vi "RFSA Configure Trigger.vi"(8 "error in (no error)":errorcluster, 11 "IVI Refnum in":refnum<k15>) -> (0 "error out":errorcluster, 3 "IVI Refnum out":refnum<k15>)   [LabVIEW 2021]
uses:
  <instrlib>/niRFSA/niRFSA.llb/niRFSA Trigger Terminals.ctl
  <instrlib>/niRFSA/niRFSA.llb/niRFSA Trigger DigEdge - Edge Values.ctl
  <instrlib>/niRFSG/niRFSG.llb/niRFSG Exported Signal Destinations.ctl
  <instrlib>/niRFSA/niRFSA.llb/niRFSA Configure Digital Edge Advance Trigger.vi
  <instrlib>/niRFSA/niRFSA.llb/niRFSA Configure Digital Edge Start Trigger.vi
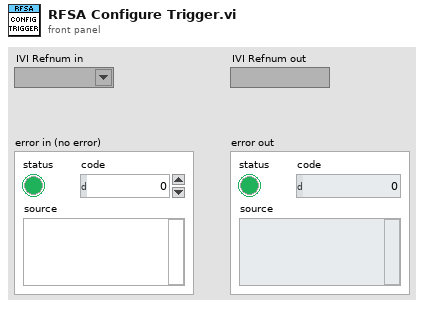
[diagram p1: front panel]
types:
  T1 = typedef "niRFSG Exported Signal Destinations.ctl" = string
  T2 = typedef "niRFSA Trigger DigEdge - Edge Values.ctl" = i32
  T3 = typedef "niRFSA Trigger Terminals.ctl" = string
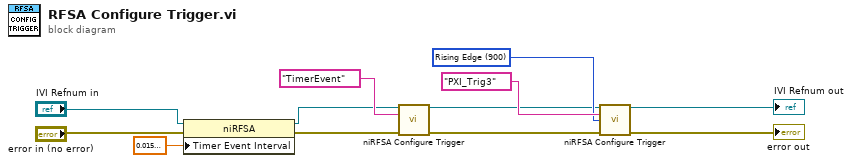
[diagram p0: block diagram]
diagram:
  w10 = T2 900 items=["Rising Edge"=900, "Falling Edge"=901] ("edge")
  n1 = property class="niRFSA"(reference="IVI Refnum in", error in="error in (no error)", "Timer Event Interval"=0.015000000000000003) -> (reference out=w1:refnum<k15>, error out=w2:errorcluster)
  n2 = call-poly <instrlib>:"niRFSA Configure Trigger.vi"("instrument handle"=w1, "source"=T3 "TimerEvent", "error in"=w2) -> ("instrument handle out"=w6:refnum<k15>, "error out"=w7:errorcluster)  [unwired: 11 in]
  n3 = call-poly <instrlib>:"niRFSA Configure Trigger.vi"("instrument handle"=w6, "source"=T1 "PXI_Trig3" ("output terminal"), "edge"=w10, "error in"=w7) -> ("instrument handle out"=→"IVI Refnum out":refnum<k15>, "error out"=→"error out":errorcluster)  [unwired: 10 in]
